vi "FiberSpectrograph_putSample_spectTemperature.vi"(8 "error in (no error)":errorcluster, 11 "spectTemperature_Ctl":T1) -> (0 "error out":errorcluster, 2 "function return":i32, 3 "spectTemperature_Ctl out":T1)   [LabVIEW 2016, in "SALLV_FiberSpectrograph.lvlib"]
doc: "int FiberSpectrograph_shm_putSample_spectTemperatureLV(FiberSpectrograph_spectTemperatureLV *spectTemperature_Ctl );"
uses:
  SALLV_FiberSpectrograph.lvlib
  DataTypes/spectTemperature.ctl
  SALLV_FiberSpectrograph.so
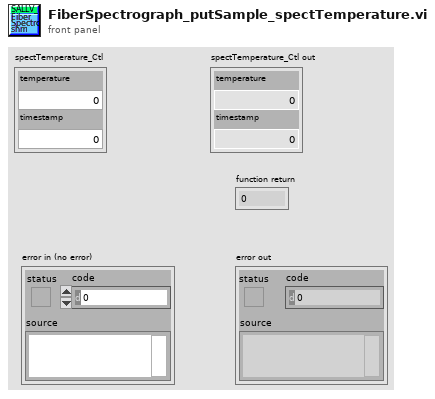
[diagram p1: front panel]
types:
  T1 = typedef "SALLV_FiberSpectrograph.lvlib/spectTemperature.ctl" = cluster{"temperature":dbl, "timestamp":dbl}
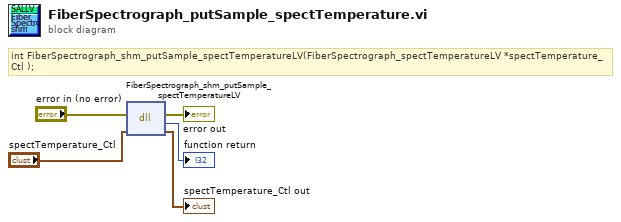
[diagram p0: block diagram]
diagram:
  # "int FiberSpectrograph_shm_putSample_spectTemperatureLV(FiberSpectrograph_spectTemperatureLV *spectTemperature_Ctl );"
  n1 = dll-call lib="home/saluser/SALLV_FiberSpectrograph/SALLV_FiberSpectrograph.*" fn="FiberSpectrograph_shm_putSample_spectTemperatureLV"(error in="error in (no error)", "spectTemperature_Ctl"="spectTemperature_Ctl") -> (error out=→"error out":errorcluster, →"function return":i32, "spectTemperature_Ctl"=→"spectTemperature_Ctl out":T1)  [unwired: 2 in, 1 out]
